vi "Write Jump Index.vi"(8 "error in (no error)":errorcluster, 10 "Jump Index":i32, 11 "Conditional Jump Step Config in":refnum<class "Conditional Jump Step Config.lvclass">) -> (0 "error out":errorcluster, 3 "Conditional Jump Step Config out":refnum<class "Conditional Jump Step Config.lvclass">)   [LabVIEW 2015, in "Conditional Jump Step Config.lvclass"]
uses:
  Conditional Jump Step Config.lvclass
  Conditional Jump Step Config.lvclass/Conditional Jump Step Config.ctl
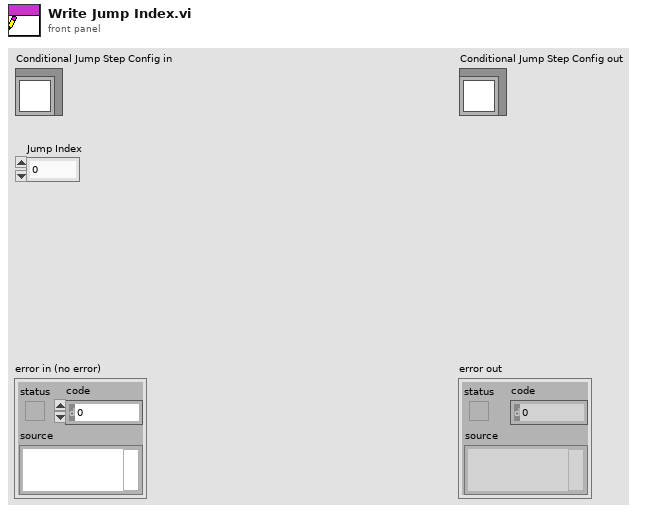
[diagram p1: front panel]
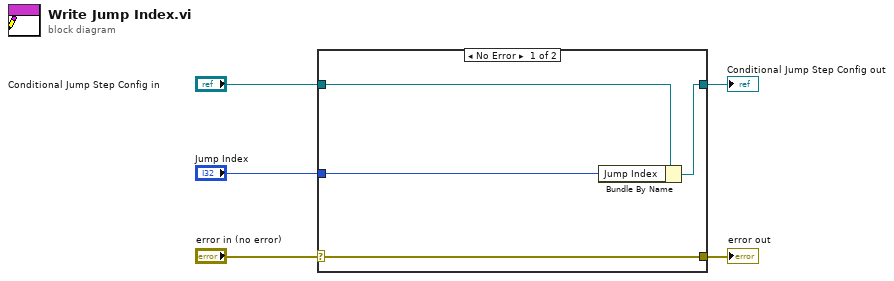
[diagram p0: block diagram]
diagram:
  n1 = case shown="No Error" "error in (no error)" {
    selector: "error in (no error)" -> [w9 w10]
    tunnel: [w9 w10] -> w4
    tunnel: [w7 w11] -> w2
    tunnel: "Conditional Jump Step Config in" -> [w8 w11]
    tunnel: "Jump Index" -> [w6 _]
    frame No Error {
      n2 = Bundle By Name(cluster=w8, "Jump Index"=w6) -> (w7:refnum<class "Conditional Jump Step Config.lvclass">)
    }
    frame Error {
    }
  }
  "error out" <- w4
  "Conditional Jump Step Config out" <- w2
